vi "ImageTrialHeaderSubVI.vi"(1 "Bytes to skip":u16, 2 "Time Stamp":timestamp format="%<%H:%M:%S%3u>T", 3 "stim number":i32, 4 "trial":u32, 5 "refnum in":refnum<file>) -> (0 "refnum out":refnum<file>)   [LabVIEW 2009]
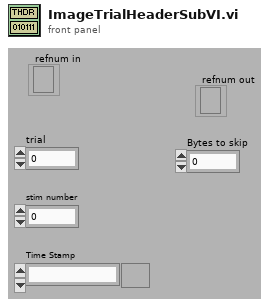
[diagram p1: front panel]
types:
  T1 = enum16{"big-endian, network order", "native, host order", "little-endian"}
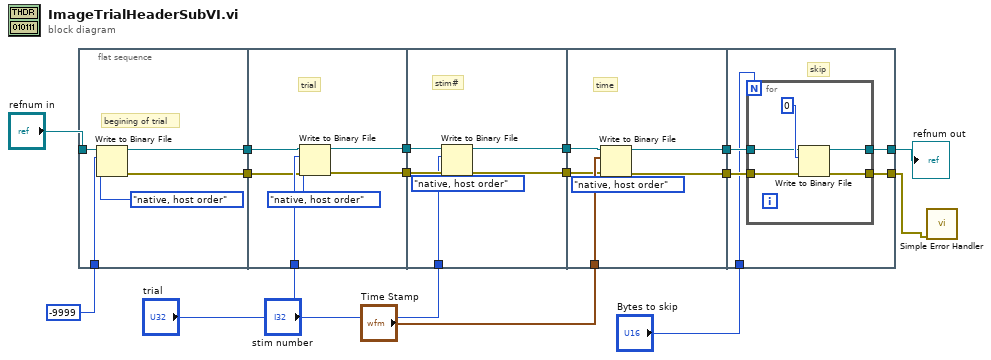
[diagram p0: block diagram]
diagram:
  n1 = flat-sequence {
    tunnel: [w21] -> w6
    tunnel: [w20] -> w5
    tunnel: -9999 -> [w19]
    tunnel: "refnum in" -> [w18]
    tunnel: "trial" -> [w27]
    tunnel: [w25] -> w16
    tunnel: [w24] -> w15
    tunnel: w6 -> [w23]
    tunnel: w5 -> [w22]
    tunnel: w16 -> [w28]
    tunnel: [w32] -> w14
    tunnel: w15 -> [w31]
    tunnel: [w30] -> w13
    tunnel: "stim number" -> [w29]
    tunnel: "Time Stamp" -> [w39]
    tunnel: w14 -> [w37]
    tunnel: [w36] -> w12
    tunnel: w13 -> [w35]
    tunnel: [w34] -> w11
    tunnel: w12 -> [w44]
    tunnel: w11 -> [w42]
    tunnel: "Bytes to skip" -> [w40]
    tunnel: [w43] -> w2
    tunnel: [w41] -> w1
    frame #0 {
      # "begining of trial"
      n2 = Write to Binary File(file (use dialog)=w18, data=w19, 9:T1."native, host order" ("byte order (0:big-endian, network order)")) -> (refnum out=w20:refnum<file>, error out=w21:errorcluster)  [unwired: 3 in, 1 out]
    }
    frame #1 {
      # "trial"
      n3 = Write to Binary File(file (use dialog)=w22, data=w27, error in=w23, 9:T1."native, host order" ("byte order (0:big-endian, network order)")) -> (refnum out=w25:refnum<file>, error out=w24:errorcluster)  [unwired: 2 in, 1 out]
    }
    frame #2 {
      # "stim#"
      n4 = Write to Binary File(file (use dialog)=w28, data=w29, error in=w31, 9:T1."native, host order" ("byte order (0:big-endian, network order)")) -> (refnum out=w32:refnum<file>, error out=w30:errorcluster)  [unwired: 2 in, 1 out]
    }
    frame #3 {
      # "time"
      n5 = Write to Binary File(file (use dialog)=w37, data=w39, error in=w35, 9:T1."native, host order" ("byte order (0:big-endian, network order)")) -> (refnum out=w36:refnum<file>, error out=w34:errorcluster)  [unwired: 2 in, 1 out]
    }
    frame #4 {
      # "skip"
      n6 = for {
        N: w40 -> [_]
        tunnel: [w49] -> w43
        tunnel: [w48] -> w41
        tunnel: w44 -> [w46]
        tunnel: w42 -> [w45]
        n7 = Write to Binary File(file (use dialog)=w46, data=i8 0, error in=w45) -> (refnum out=w49:refnum<file>, error out=w48:errorcluster)  [unwired: 3 in, 1 out]
      }
    }
  }
  n8 = call <vilib>:"Simple Error Handler.vi"("error in (no error)"=w1) -> ()  [unwired: 4 in, 5 out]
  "refnum out" <- w2
